vi "Fit Transform.vi"(8 "error in (no error)":errorcluster caption="entrée d'erreur (pas d'erreur)", 9 "doc":string, 10 "X":string[][](array[string]), 11 "HashingVectorizer.lvclass":refnum<class "HashingVectorizer.lvclass">) -> (0 "error out":errorcluster caption="sortie d'erreur", 2 "Data":T1, 3 "HashingVectorizer.lvclass":refnum<class "HashingVectorizer.lvclass">)   [LabVIEW 2020, in "HashingVectorizer.lvclass"]
doc: "Transform a sequence of documents to a document-term matrix.\n\nReturns : \n\n- X : sparse matrix of shape (n_samples, n_features)\nDocument-term matrix."
uses:
  HashingVectorizer.lvclass
  HashingVectorizer.lvclass/HashingVectorizer.ctl
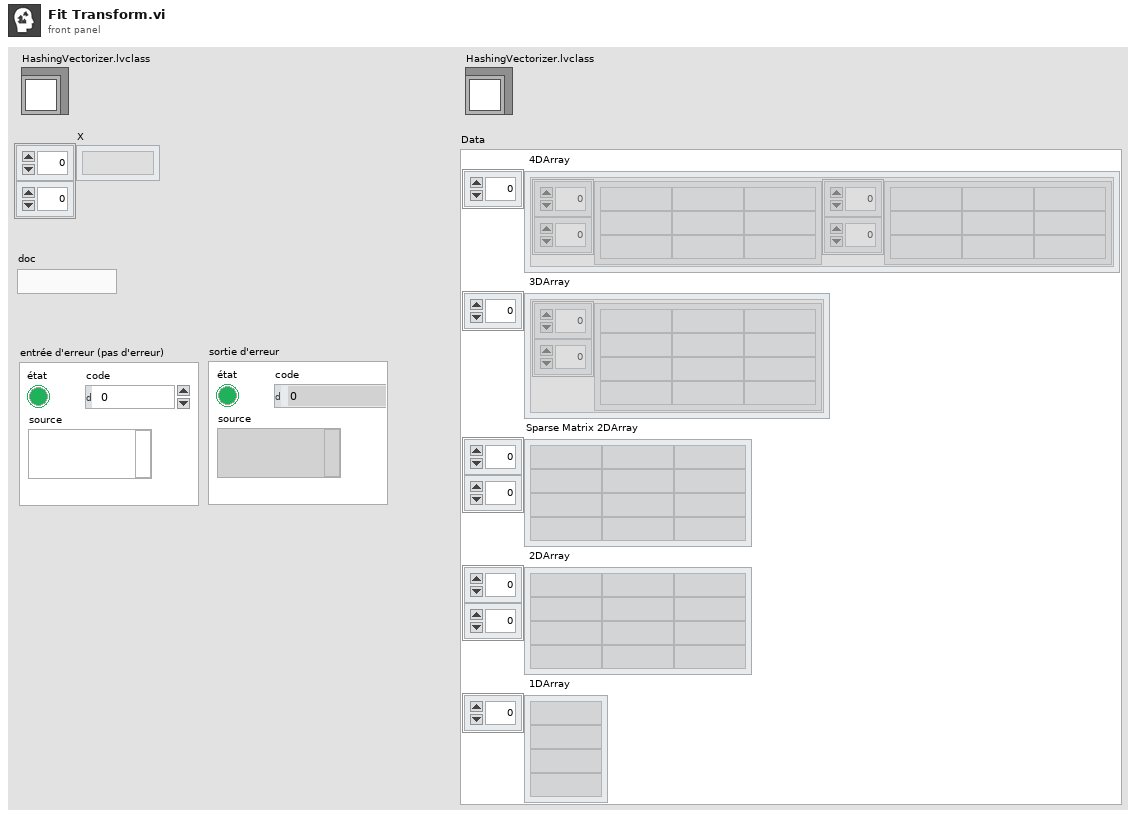
[diagram p1: front panel]
types:
  T1 = cluster{" 4DArray":cluster{"1":string[][], "2":string[][]}[], " 3DArray":cluster{"Tableau":string[][]}[], "Sparse Matrix 2DArray":string[][], " 2DArray":string[][], " 1DArray":string[]}
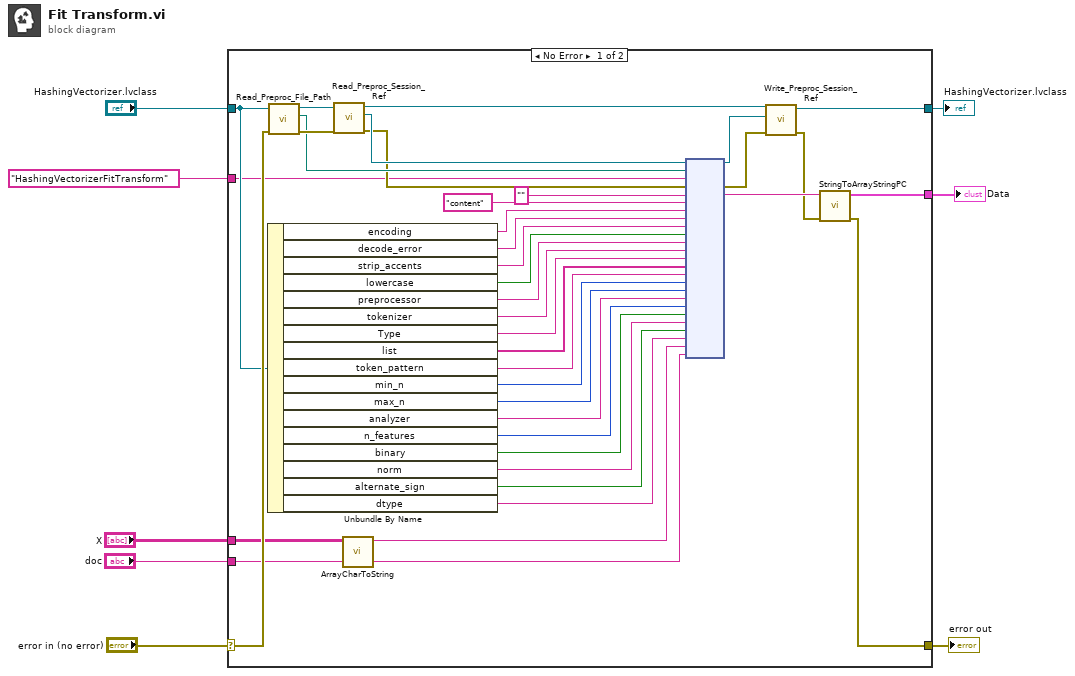
[diagram p0: block diagram]
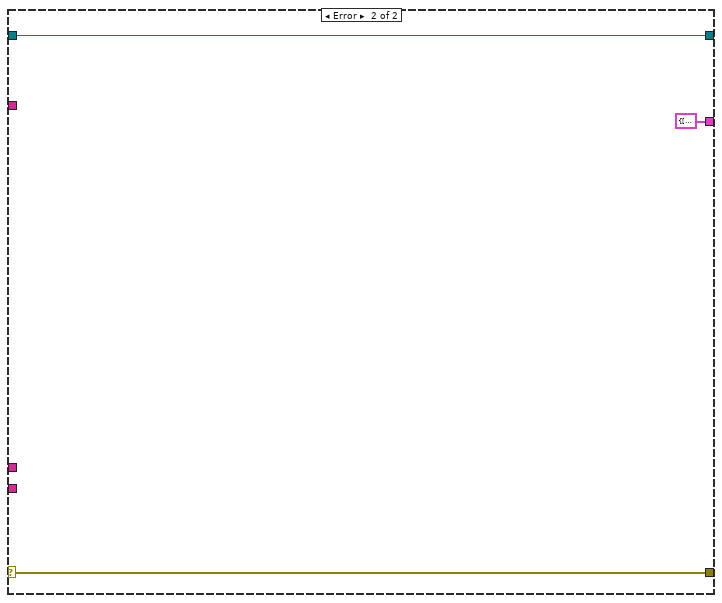
[diagram p2: hidden frame]
diagram:
  n1 = case shown="No Error" "error in (no error)" {
    selector: "error in (no error)" -> [w35 w49]
    tunnel: [w9 w49] -> w7
    tunnel: [w13 w48] -> w5
    tunnel: "HashingVectorizer.lvclass" -> [w34 w48]
    tunnel: "HashingVectorizerFitTransform" ("Fonction") -> [w33 _]
    tunnel: [w10 T1 {" 4DArray"=[], " 3DArray"=[], "Sparse Matrix 2DArray"=[], " 2DArray"=[], " 1DArray"=[]} ("Data")] -> w1
    tunnel: "X" -> [w15 _]
    tunnel: "doc" -> [w16 _]
    frame No Error {
      n2 = Unbundle By Name(w34) -> ("encoding"=w37:string, "decode_error"=w36:string, "strip_accents"=w32:string, "lowercase"=w31:bool, "preprocessor"=w30:string, "tokenizer"=w29:string, "Type"=w27:string, "list"=w26:string[], "token_pattern"=w25:string, "min_n"=w24:i32, "max_n"=w23:i32, "analyzer"=w22:string, "n_features"=w21:i32, "binary"=w20:bool, "norm"=w19:string, "alternate_sign"=w18:bool, "dtype"=w17:string)
      n3 = call-dynamic "Read_Preproc_File_Path.vi"("error in (no error)"=w35, "Python in"=w34) -> ("error out"=w45:errorcluster, "File_Path"=w44:path, "Python out"=w46:refnum<class "HashingVectorizer.lvclass">)  [unwired: 7 in]
      n4 = call-dynamic "Read_Preproc_Session_Ref.vi"("error in (no error)"=w45, "Python in"=w46) -> ("error out"=w42:errorcluster, "Session_ref"=w43:refnum<k35>, "Python out"=w41:refnum<class "HashingVectorizer.lvclass">)  [unwired: 7 in]
      n5 = call "ArrayCharToString.vi"("TAB"=w15) -> ("Instruction"=w14:string)  [unwired: 10 in]
      n6 = node(w43, w44, w33, w42, "", "content", w37, w36, w32, w31, w30, w29, w27, w26, w25, w24, w23, w22, w21, w20, w19, w18, w17, w14, w16) -> (w39:refnum<k35>, w40:errorcluster, w12:string)  [unwired: 20 in, 2 out]
      n7 = call-dynamic "Write_Preproc_Session_Ref.vi"("error in (no error)"=w40, "Session_ref"=w39, "Python in"=w41) -> ("error out"=w11:errorcluster, "Python out"=w13:refnum<class "HashingVectorizer.lvclass">)  [unwired: 7 in]
      n8 = call "StringToArrayStringPC.vi"("sortie d'erreur"=w11, "Return value"=w12) -> ("sortie d'erreur"=w9:errorcluster, "Data"=w10:T1)  [unwired: 8 in]
    }
    frame Error {
    }
  }
  "error out" <- w7
  "HashingVectorizer.lvclass" <- w5
  "Data" <- w1
